vi "build.vi"(8 "error in (no error)":errorcluster, 11 "FrameBuilder in":refnum<class "FrameBuilder.lvclass">) -> (0 "error out":errorcluster, 2 "Frame":T1 {"Data" format="%02x"}, 3 "FrameBuilder out":refnum<class "FrameBuilder.lvclass">)   [LabVIEW 2015, in "FrameBuilder.lvclass"]
uses:
  FrameBuilder.lvclass
  Typedefs/Frame.ctl
  FrameBuilder.lvclass/FrameBuilder.ctl
  Typedefs/RTTypeDefs.lvlib
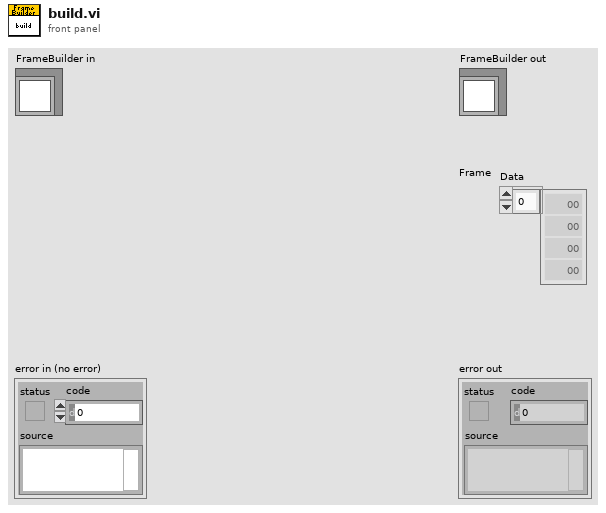
[diagram p1: front panel]
types:
  T1 = typedef "RTTypeDefs.lvlib/Frame.ctl" = cluster{"Data":u8[]}
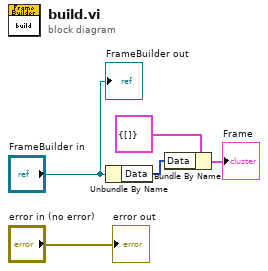
[diagram p0: block diagram]
diagram:
  n1 = Unbundle By Name("FrameBuilder in") -> ("Data"=w3:u8[])
  n2 = Bundle By Name(cluster=T1 {"Data"=[]} ("Frame"), "Data"=w3) -> (→"Frame":T1)
  "error out" <- "error in (no error)"
  "FrameBuilder out" <- "FrameBuilder in"
